vi "Measure.vi"(8 "error in":errorcluster, 11 "SwitchMatrix in":refnum<class "SwitchMatrix.lvclass">) -> (0 "error out":errorcluster, 3 "SwitchMatrix out":refnum<class "SwitchMatrix.lvclass">)   [LabVIEW 2019, in "SwitchMatrix.lvlib" / "SwitchMatrix.lvclass"]
uses:
  Library/SwitchMatrix.lvclass
  builds/Instruments/Instruments.lvlibp/Library/Instruments.lvclass
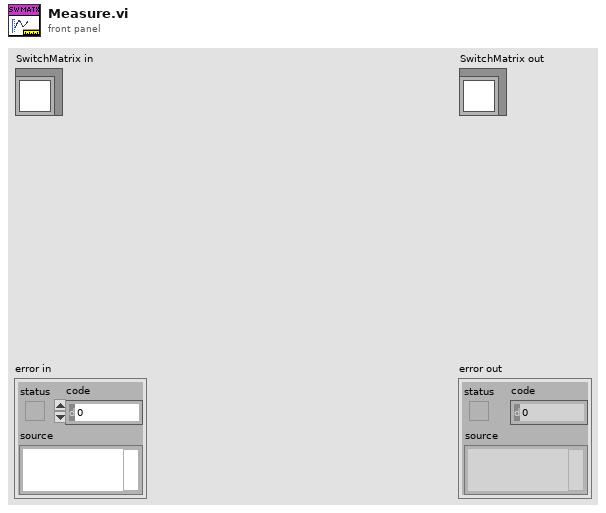
[diagram p1: front panel]
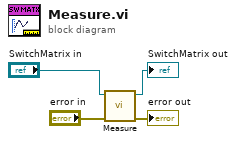
[diagram p0: block diagram]
diagram:
  n1 = call-parent "Measure.vi"("error in"="error in", "Instruments in"="SwitchMatrix in") -> ("error out"=→"error out":errorcluster, "Instruments out"=→"SwitchMatrix out":refnum<class "SwitchMatrix.lvclass">)  [unwired: 8 in]
